vi "探头启用设置.vi"() -> ()   [LabVIEW 2016, in "斯坦道多参数.lvlib"]
uses:
  <vilib>/Utility/miscctls.llb/LVPointTypeDef.ctl
panel:
  in  "水中油启用":bool
  in  "氨氮启用":bool
  in  "氯化物启用":bool
  in  "藻密度单位":enum16{"cells/mL", "cells/L"}(ring)
  in  "叶绿素a单位":enum16{"μg/L", "mg/L"}(ring)
  in  "关闭":bool
  in  "水温通道":u16(ring)=1 items=["pH", "DO", "浊度", "电导率", "叶绿素a", "藻密度"]
  in  "DO2探头选择":T1=enum."国弘"
  in  "DO2启用":bool
  in  "COD探头选择":T1=enum."国弘"
  in  "COD启用":bool
  in  "pH":bool
  in  "DO":bool
  in  "Turb":bool
  in  "Cond":bool
  in  "Temp":bool
  in  "叶绿素a启用":bool
  in  "藻密度":bool
  in  "pH探头选择":T1
  in  "DO探头选择":T1
  in  "电导率探头选择":T1
  in  "浊度探头选择":T1
  in  "叶绿素a探头选择":T1
  in  "藻密度探头选择":T1
  in  "ORP启用":bool
  in  "ORP探头选择":T1
  # "请选择要启用的参数"
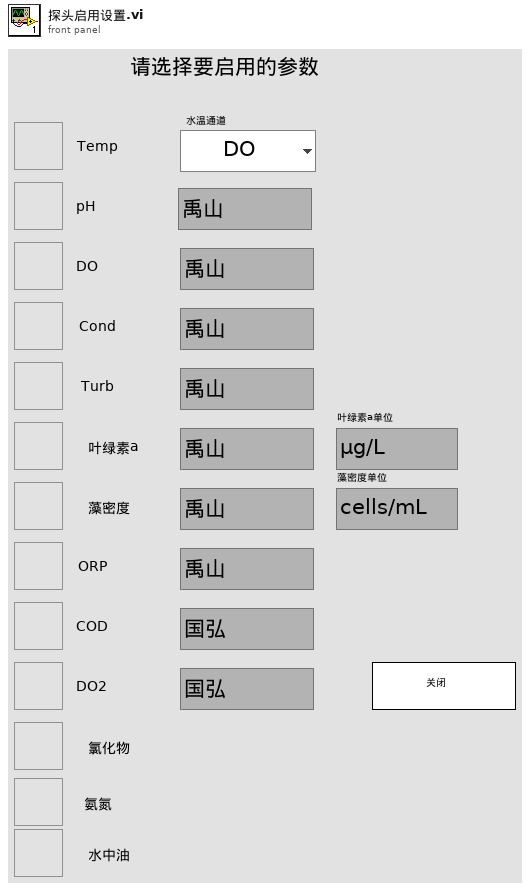
[diagram p1: front panel]
types:
  T1 = typedef "斯坦道多参数.lvlib/探头类型.ctl" = enum16{"禹山", "国弘", "纳清", "STD"}
  T2 = typedef "LVPointTypeDef.ctl" = cluster{"Horizontal":i16, "Vertical":i16}
  T3 = cluster{"pH探头选择":T1, "DO探头选择":T1, "电导率探头选择":T1, "浊度探头选择":T1, "叶绿素a探头选择":T1, "蓝绿藻探头选择":T1, "orp探头选择":T1, "COD探头选择":T1, "DO2探头选择":T1, "氨氮探头选择":T1, "水中油探头选择":T1}
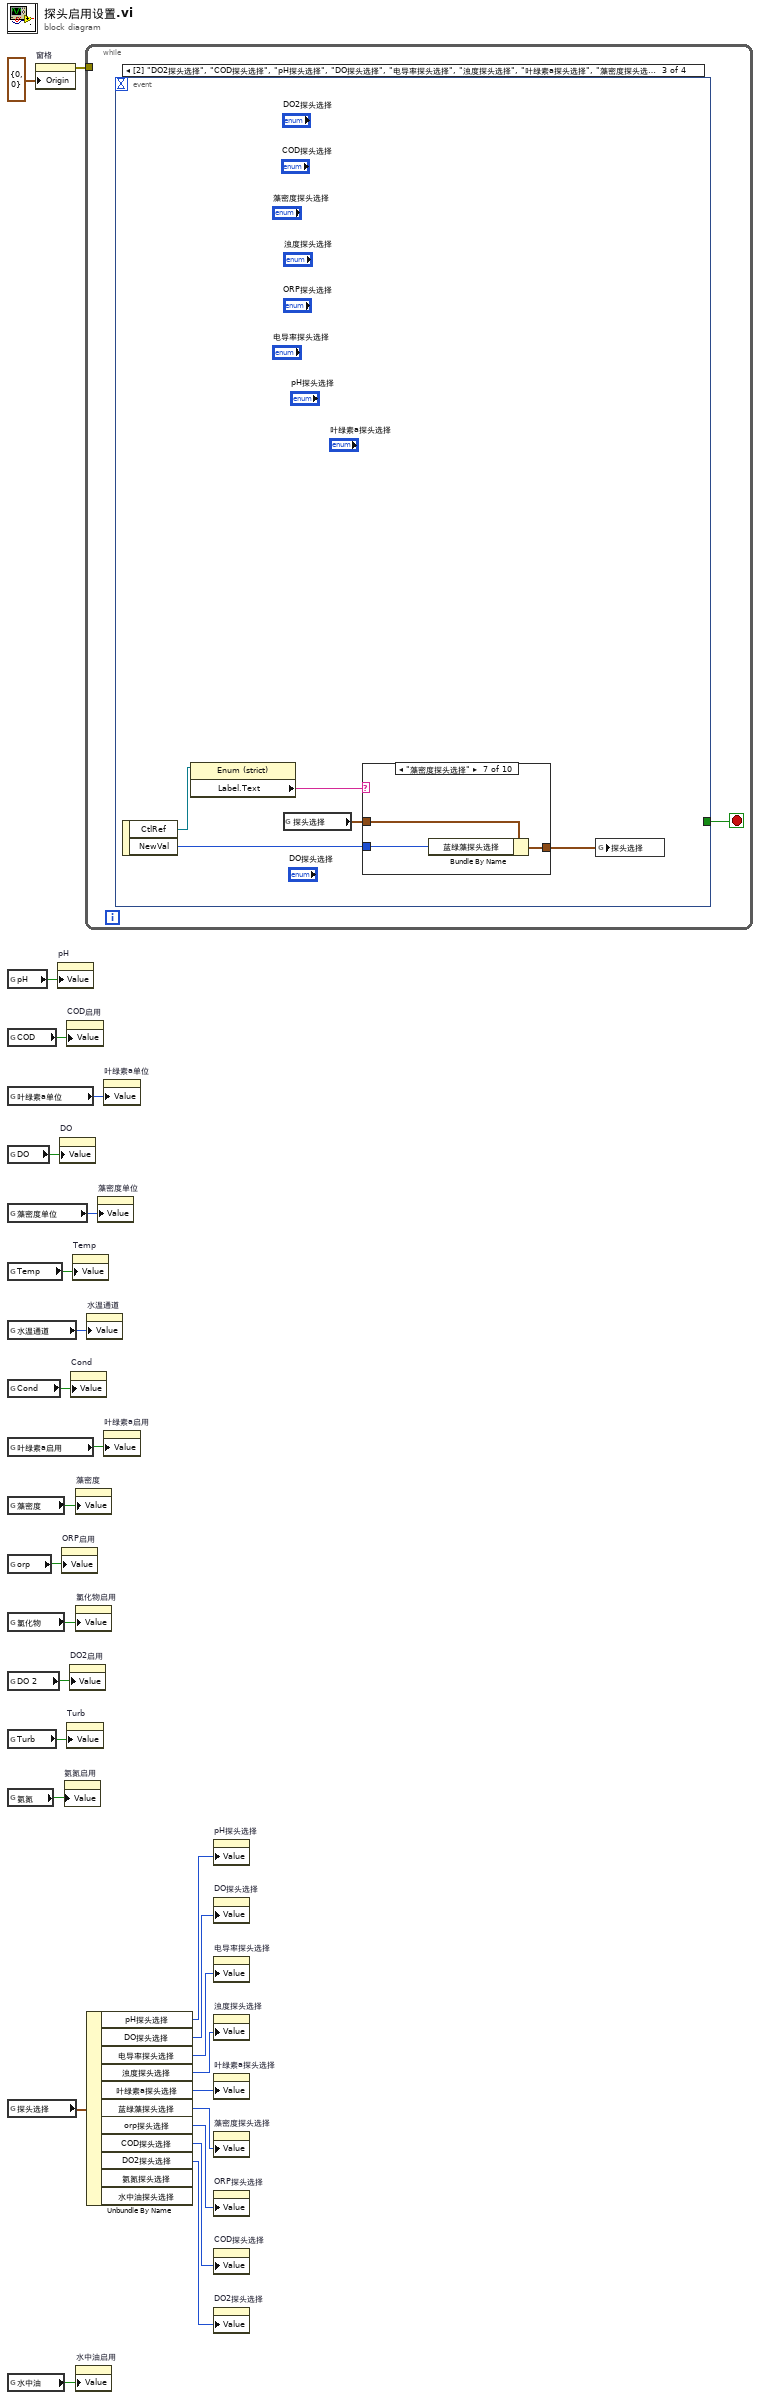
[diagram p0: block diagram]
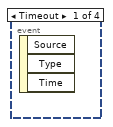
[diagram p2: hidden frame]
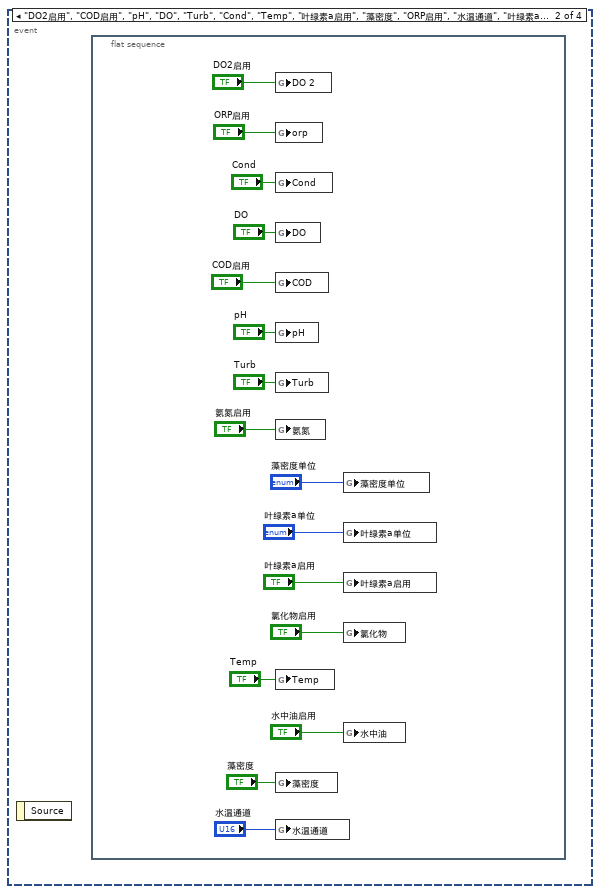
[diagram p3: hidden frame]
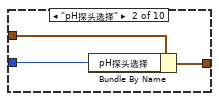
[diagram p5: hidden frame]
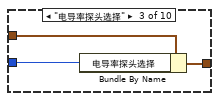
[diagram p6: hidden frame]
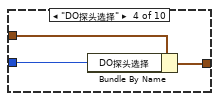
[diagram p7: hidden frame]
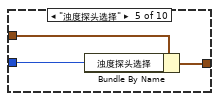
[diagram p8: hidden frame]
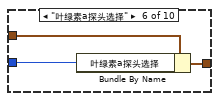
[diagram p9: hidden frame]
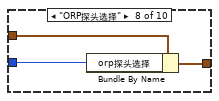
[diagram p10: hidden frame]
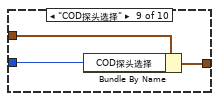
[diagram p11: hidden frame]
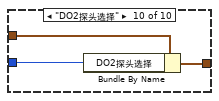
[diagram p12: hidden frame]
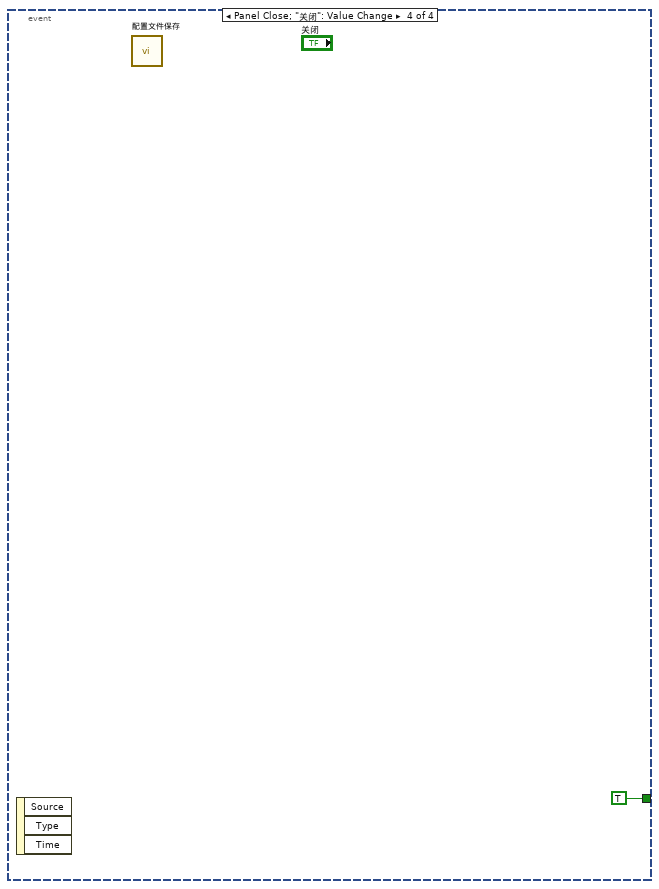
[diagram p13: hidden frame]
diagram:
  n1 = global read "断电保存变量.vi" "pH"() -> (w26:bool)
  n2 = global read "断电保存变量.vi" "COD"() -> (w25:bool)
  n3 = global read "断电保存变量.vi" "叶绿素a单位"() -> (w5:enum16{"μg/L", "mg/L"})
  n4 = global read "断电保存变量.vi" "DO"() -> (w24:bool)
  n5 = global read "断电保存变量.vi" "藻密度单位"() -> (w6:enum16{"cells/mL", "cells/L"})
  n6 = global read "断电保存变量.vi" "Temp"() -> (w23:bool)
  n7 = global read "断电保存变量.vi" "水温通道"() -> (w22:enum16{"pH", "DO", "浊度", "电导率", "叶绿素a", "藻密度"})
  n8 = global read "断电保存变量.vi" "Cond"() -> (w21:bool)
  n9 = global read "断电保存变量.vi" "叶绿素a启用"() -> (w20:bool)
  n10 = global read "断电保存变量.vi" "藻密度"() -> (w19:bool)
  n11 = global read "断电保存变量.vi" "orp"() -> (w18:bool)
  n12 = global read "断电保存变量.vi" "氯化物"() -> (w4:bool)
  n13 = global read "断电保存变量.vi" "DO 2"() -> (w17:bool)
  n14 = global read "断电保存变量.vi" "Turb"() -> (w16:bool)
  n15 = global read "断电保存变量.vi" "氨氮"() -> (w3:bool)
  n16 = global read "断电保存变量.vi" "探头选择"() -> (w15:T3)
  n17 = global read "断电保存变量.vi" "水中油"() -> (w2:bool)
  n18 = property on="窗格" class="Pane"("Origin"=T2 {"Horizontal"=0, "Vertical"=0} ("原点")) -> (error out=w27:errorcluster)  [unwired: 2 in, 1 out]
  n19 = property on="pH" class="Bool (strict)"("Value"=w26) -> ()  [unwired: 2 in, 2 out]
  n20 = property on="DO" class="Bool (strict)"("Value"=w24) -> ()  [unwired: 2 in, 2 out]
  n21 = property on="ORP启用" class="Bool (strict)"("Value"=w18) -> ()  [unwired: 2 in, 2 out]
  n22 = property on="氨氮启用" class="Bool (strict)"("Value"=w3) -> ()  [unwired: 2 in, 2 out]
  n23 = property on="COD启用" class="Bool (strict)"("Value"=w25) -> ()  [unwired: 2 in, 2 out]
  n24 = property on="Turb" class="Bool (strict)"("Value"=w16) -> ()  [unwired: 2 in, 2 out]
  n25 = property on="DO2启用" class="Bool (strict)"("Value"=w17) -> ()  [unwired: 2 in, 2 out]
  n26 = property on="Cond" class="Bool (strict)"("Value"=w21) -> ()  [unwired: 2 in, 2 out]
  n27 = property on="Temp" class="Bool (strict)"("Value"=w23) -> ()  [unwired: 2 in, 2 out]
  n28 = property on="藻密度" class="Bool (strict)"("Value"=w19) -> ()  [unwired: 2 in, 2 out]
  n29 = property on="氯化物启用" class="Bool (strict)"("Value"=w4) -> ()  [unwired: 2 in, 2 out]
  n30 = property on="水中油启用" class="Bool (strict)"("Value"=w2) -> ()  [unwired: 2 in, 2 out]
  n31 = while {
    tunnel: w27 -> [_]
    stop <- w29 stop-if-true
    n32 = event shown="[2] \"DO2探头选择\", \"COD探头选择\", \"pH探头选择\", \"DO探头选择\", \"电导率探头选择\", \"浊度探头选择\", \"叶绿素a探头选择\", \"藻密度探头选择\", \"ORP探头选择\": Value Change" {
      selector: _ -> [_ _ _ _]
      dyn-events: _ -> [_ _ _ _]
      timeout: _ -> [_ _ _ _]
      tunnel: [_ _ _ TRUE] -> w29
      event Timeout {
        n33 = event-data() -> ()  [unwired: 1 in, 3 out]
      }
      event "DO2启用", "COD启用", "pH", "DO", "Turb", "Cond", "Temp", "叶绿素a启用", "藻密度", "ORP启用", "水温通道", "叶绿素a单位", "藻密度单位", "氯化物启用", "氨氮启用", "水中油启用": Value Change {
        n34 = event-data() -> ()  [unwired: 1 in, 1 out]
        n35 = flat-sequence {
          frame #0 {
            n36 = global write "断电保存变量.vi" "DO 2"("DO2启用") -> ()
            n37 = global write "断电保存变量.vi" "orp"("ORP启用") -> ()
            n38 = global write "断电保存变量.vi" "Cond"("Cond") -> ()
            n39 = global write "断电保存变量.vi" "DO"("DO") -> ()
            n40 = global write "断电保存变量.vi" "COD"("COD启用") -> ()
            n41 = global write "断电保存变量.vi" "pH"("pH") -> ()
            n42 = global write "断电保存变量.vi" "Turb"("Turb") -> ()
            n43 = global write "断电保存变量.vi" "氨氮"("氨氮启用") -> ()
            n44 = global write "断电保存变量.vi" "Temp"("Temp") -> ()
            n45 = global write "断电保存变量.vi" "藻密度"("藻密度") -> ()
            n46 = global write "断电保存变量.vi" "水温通道"("水温通道") -> ()
            n47 = global write "断电保存变量.vi" "藻密度单位"("藻密度单位") -> ()
            n48 = global write "断电保存变量.vi" "叶绿素a单位"("叶绿素a单位") -> ()
            n49 = global write "断电保存变量.vi" "叶绿素a启用"("叶绿素a启用") -> ()
            n50 = global write "断电保存变量.vi" "氯化物"("氯化物启用") -> ()
            n51 = global write "断电保存变量.vi" "水中油"("水中油启用") -> ()
          }
        }
      }
      event Value Change {
        n52 = event-data() -> ("CtlRef"=w47:refnum<vi>, "NewVal"=w46:T1)  [unwired: 1 in]
        n53 = property class="Enum (strict)"(reference=w47) -> ("Label.Text"=w50:string)  [unwired: 1 in, 2 out]
        n54 = global read "断电保存变量.vi" "探头选择"() -> (w49:T3)
        n55 = case shown="\"藻密度探头选择\"" w50 {
          tunnel: w49 -> [w51 w54 w57 w60 w63 w66 w69 w72 w75 w78]
          tunnel: [w51 w53 w56 w59 w62 w65 w68 w71 w74 w77] -> w48
          tunnel: w46 -> [_ w52 w55 w58 w61 w64 w67 w70 w73 w76]
          frame Default {
          }
          frame "pH探头选择" {
            n56 = Bundle By Name(cluster=w54, "pH探头选择"=w52) -> (w53:T3)
          }
          frame "电导率探头选择" {
            n57 = Bundle By Name(cluster=w57, "电导率探头选择"=w55) -> (w56:T3)
          }
          frame "DO探头选择" {
            n58 = Bundle By Name(cluster=w60, "DO探头选择"=w58) -> (w59:T3)
          }
          frame "浊度探头选择" {
            n59 = Bundle By Name(cluster=w63, "浊度探头选择"=w61) -> (w62:T3)
          }
          frame "叶绿素a探头选择" {
            n60 = Bundle By Name(cluster=w66, "叶绿素a探头选择"=w64) -> (w65:T3)
          }
          frame "藻密度探头选择" {
            n61 = Bundle By Name(cluster=w69, "蓝绿藻探头选择"=w67) -> (w68:T3)
          }
          frame "ORP探头选择" {
            n62 = Bundle By Name(cluster=w72, "orp探头选择"=w70) -> (w71:T3)
          }
          frame "COD探头选择" {
            n63 = Bundle By Name(cluster=w75, "COD探头选择"=w73) -> (w74:T3)
          }
          frame "DO2探头选择" {
            n64 = Bundle By Name(cluster=w78, "DO2探头选择"=w76) -> (w77:T3)
          }
        }
        n65 = global write "断电保存变量.vi" "探头选择"(w48) -> ()
      }
      event Panel Close; "关闭": Value Change {
        n66 = event-data() -> ()  [unwired: 1 in, 3 out]
        n67 = call "配置文件保存.vi"() -> ()  [unwired: 12 in]
      }
    }
  }
  n68 = property on="水温通道" class="Ring (strict)"("Value"=w22) -> ()  [unwired: 2 in, 2 out]
  n69 = Unbundle By Name(w15) -> ("pH探头选择"=w1:T1, "DO探头选择"=w14:T1, "电导率探头选择"=w13:T1, "浊度探头选择"=w12:T1, "叶绿素a探头选择"=w11:T1, "蓝绿藻探头选择"=w10:T1, "orp探头选择"=w9:T1, "COD探头选择"=w8:T1, "DO2探头选择"=w7:T1)  [unwired: 2 out]
  n70 = property on="藻密度单位" class="Enum (strict)"("Value"=w6) -> ()  [unwired: 2 in, 2 out]
  n71 = property on="叶绿素a单位" class="Enum (strict)"("Value"=w5) -> ()  [unwired: 2 in, 2 out]
  n72 = property on="叶绿素a启用" class="Bool (strict)"("Value"=w20) -> ()  [unwired: 2 in, 2 out]
  n73 = property on="pH探头选择" class="Enum (strict)"("Value"=w1) -> ()  [unwired: 2 in, 2 out]
  n74 = property on="DO探头选择" class="Enum (strict)"("Value"=w14) -> ()  [unwired: 2 in, 2 out]
  n75 = property on="电导率探头选择" class="Enum (strict)"("Value"=w13) -> ()  [unwired: 2 in, 2 out]
  n76 = property on="浊度探头选择" class="Enum (strict)"("Value"=w12) -> ()  [unwired: 2 in, 2 out]
  n77 = property on="叶绿素a探头选择" class="Enum (strict)"("Value"=w11) -> ()  [unwired: 2 in, 2 out]
  n78 = property on="藻密度探头选择" class="Enum (strict)"("Value"=w10) -> ()  [unwired: 2 in, 2 out]
  n79 = property on="ORP探头选择" class="Enum (strict)"("Value"=w9) -> ()  [unwired: 2 in, 2 out]
  n80 = property on="COD探头选择" class="Enum (strict)"("Value"=w8) -> ()  [unwired: 2 in, 2 out]
  n81 = property on="DO2探头选择" class="Enum (strict)"("Value"=w7) -> ()  [unwired: 2 in, 2 out]
